vi "initialize for local run.vi"(8 "error in":errorcluster, 10 "size (1,10000)":i32=1000, 11 "communicator in":refnum<class "communicator.lvclass">) -> (0 "error out":errorcluster, 3 "communicator out":refnum<class "communicator.lvclass">)   [LabVIEW 2015, in "communicator.lvclass"]
uses:
  communicator.lvclass
  communicator.lvclass/communicator.ctl
  communicator queue/identifying queue.lvclass
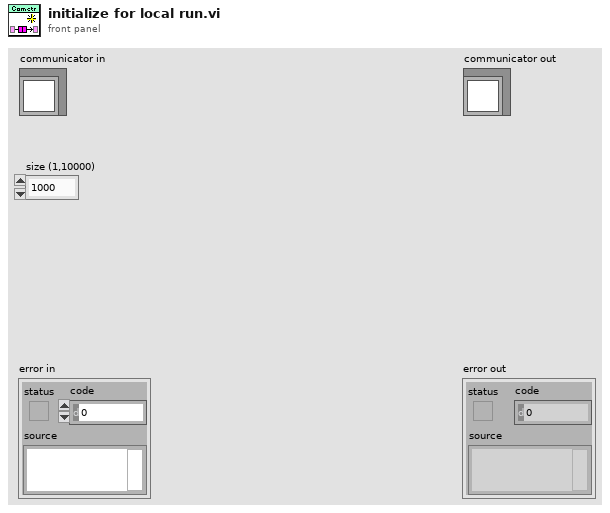
[diagram p1: front panel]
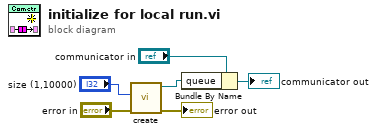
[diagram p0: block diagram]
diagram:
  n1 = call "create.vi"("error in"="error in", "size (1,10000)"="size (1,10000)") -> ("error out"=→"error out":errorcluster, "message connection out"=w2:refnum<class "identifying queue.lvclass">)  [unwired: 8 in]
  n2 = Bundle By Name(cluster="communicator in", "queue"=w2) -> (→"communicator out":refnum<class "communicator.lvclass">)
